vi "RT Main 9049.vi"() -> ()   [LabVIEW 2018]
doc: "This template is for the Queued Message Handler design pattern.\n\nThe Event Handling Loop generates messages based on user interface actions.\n\nThe Message Handling Loop processes messages generated by the Event Handling Loop, or by other messages. The messages are string values, so new messages can be added easily to the Message Cases case structure in the Message Handling Loop. Each message cluster can also provide an optional value for Message Data, which is a variant that can be converted to whatever message-specific data is required."
uses:
  support/Message Queue/Message Queue.lvlib
  Globals/Global - All RT Loop Stop.vi
  Globals/Global - Configuration Options.vi
  <vilib>/rvi/interface/nirviCloseFPGA/nirviCloseFPGA.xnode
  Globals/Global - RT Stream Connections.vi
  <vilib>/nisyscfg/nisyscfg.lvlib
  COMET  Extra Programs/Globals/Global - Monitoring Variables.vi
  controls/FPGA VI Reference 9049.ctl
  <vilib>/FPGAPlugInAG/Dynamic/niLvFpga_Close_Dynamic.vi
panel:
  out "error out":errorcluster
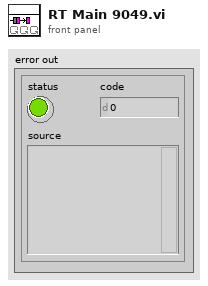
[diagram p1: front panel]
types:
  T1 = typedef "Acquisition and Logging Configuration.ctl" = cluster{"Samples per Read 9237":i32, "Number of Reads to Save":i32, "Data File Name 9222_9039_EXP":string, "TDMS Properties 9222":T2[], "Number of Channels 9237_9049_MAIN":i32, "Trigger - RMS Value":dbl, "Trigger - Channel":i32, "Trigger - Time (Minute)":i32, "Data Rate 9237":T3, "Number of Channels 9222_9039_EXP":i32, "Samples per Read 9222":i32, "Data Rate 9222":i32, "Channel Names 9222_9039_EXP":string[], "TDMS Properties 9237":T2[], "Data File Name 9237_9049":string, "Excitation Voltage":T4, "Data File Name 9222_9049_MAIN":string, "Number of Channels 9222_9049_MAIN":i32, "Channel Names 9222_9049_MAIN":string[], "Data File Name 9237_9039":string, "Channel Names 9237_9039_EXP":string[], "Channel Names 9237_9049_MAIN":string[], "Number of Channels 9237_9039_EXP":i32}
  T2 = typedef "TDMS Properties.ctl" = cluster{"Name":string, "Value":string}
  T3 = typedef "nicrio_cRIO-9237_DataRatesRing.ctl" = u8
  T4 = typedef "nicrio_cRIO-9237_ExcitationVoltageRing.ctl" = u8
  T5 = typedef "FPGA VI Reference 9049.ctl" = refnum<k20>
  T6 = typedef "Message Queue.lvlib/All Real-Time Message Queues Multi Queues.ctl" = cluster{"Message Handler":refnum<queue>, "Acquisition and Logging 9237":refnum<queue>, "Emergeny Stop for DCs":refnum<queue>, "LNG DC Commands":refnum<queue>, "LOX DC Commands":refnum<queue>, "NGV DC Commands":refnum<queue>, "Acquisition and Logging 9222":refnum<queue>, "Acquisition and Logging 9222_MAIN":refnum<queue>, "AUTO P&D":refnum<queue>, "Pressure Control":refnum<queue>}
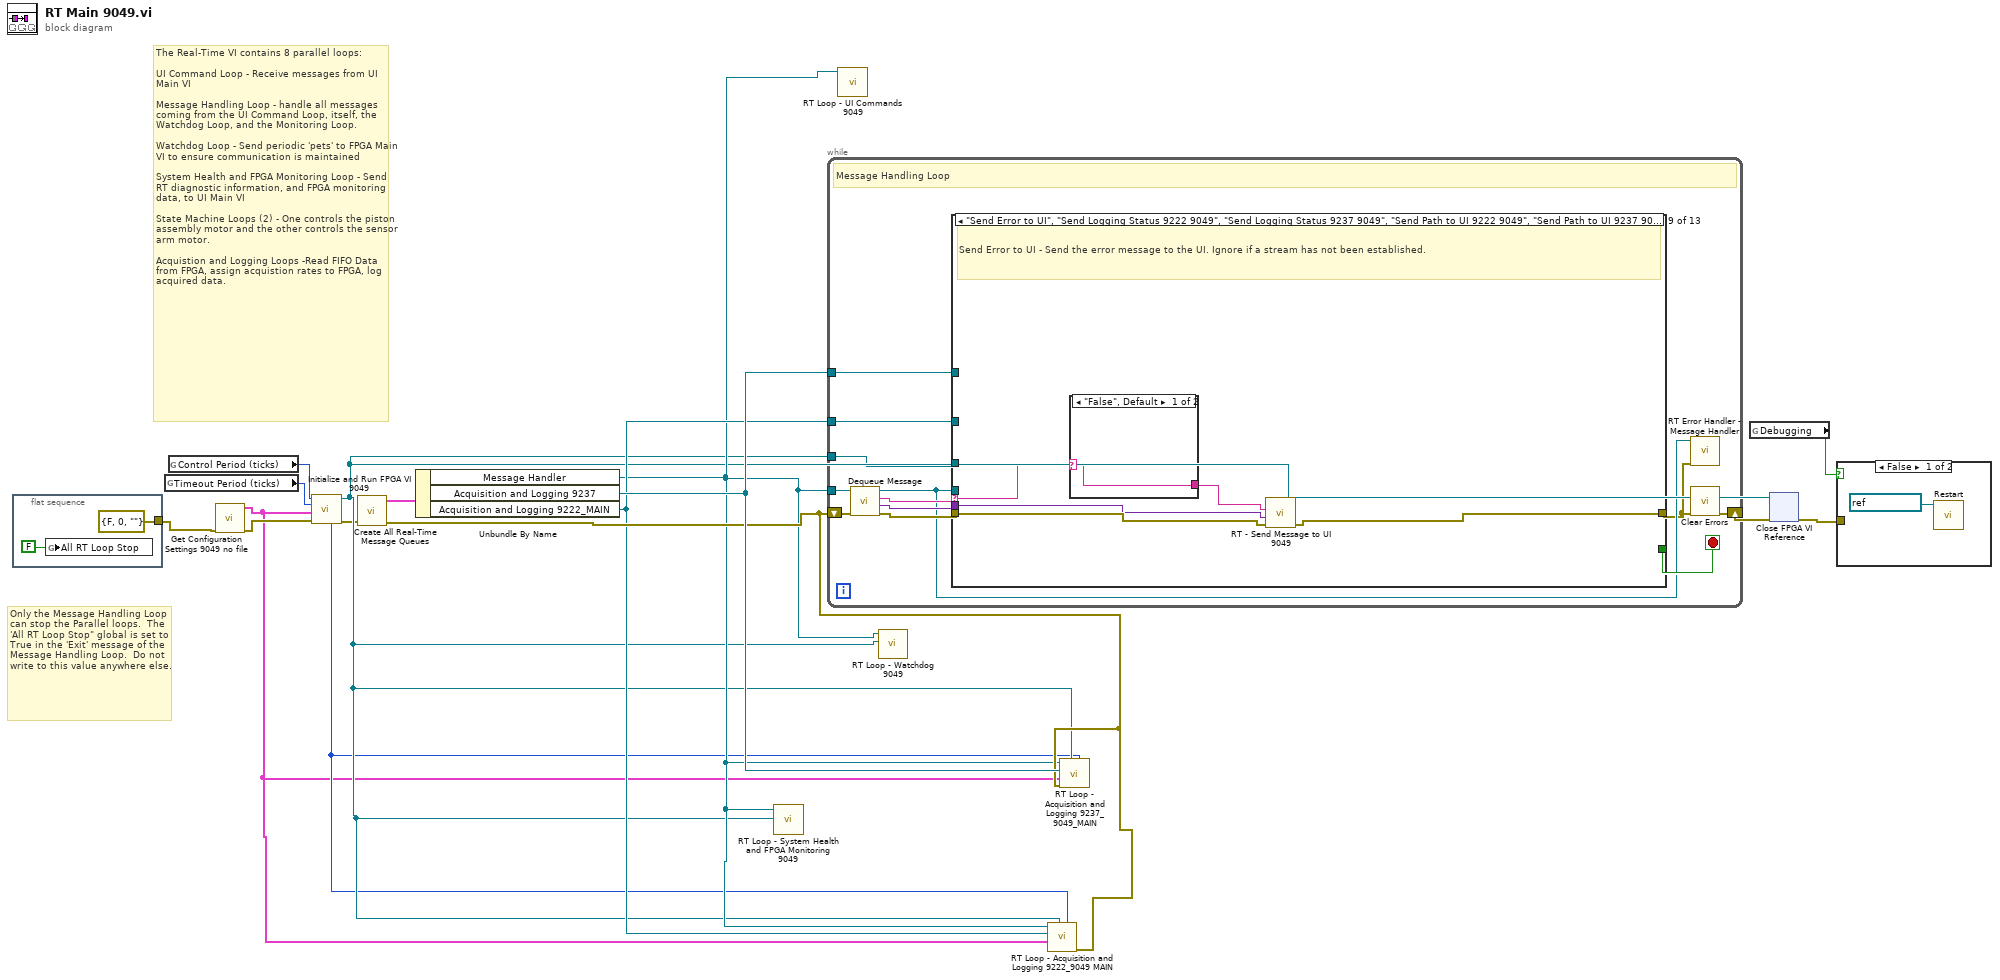
[diagram p0: block diagram]
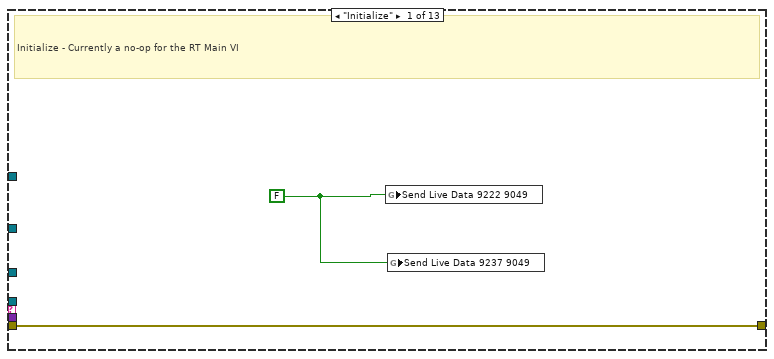
[diagram p3: hidden frame]
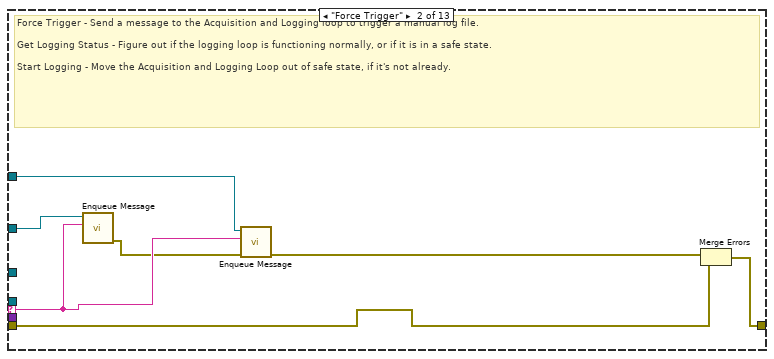
[diagram p4: hidden frame]
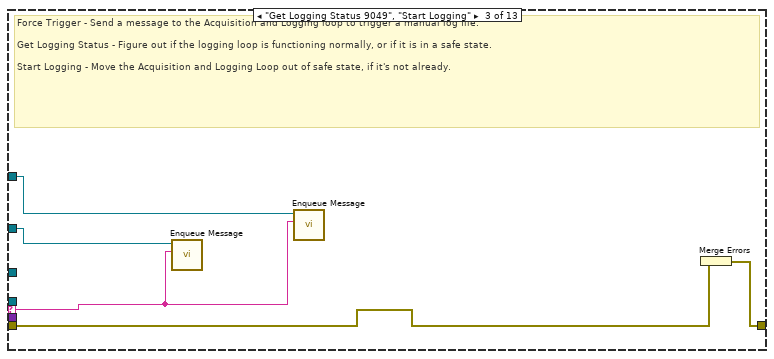
[diagram p5: hidden frame]
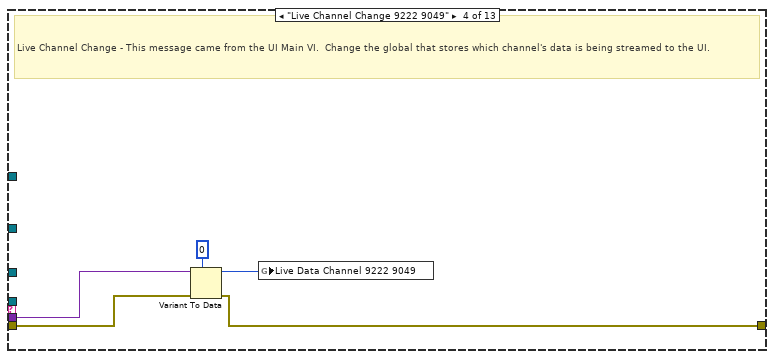
[diagram p6: hidden frame]
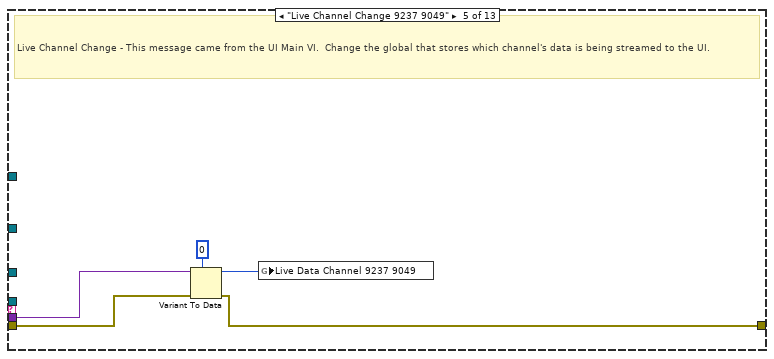
[diagram p7: hidden frame]
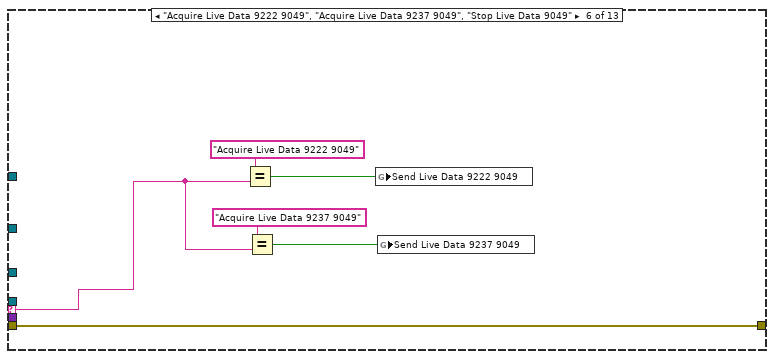
[diagram p8: hidden frame]
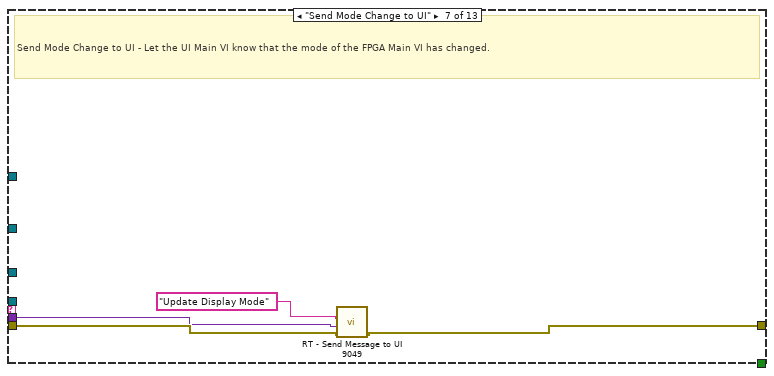
[diagram p9: hidden frame]
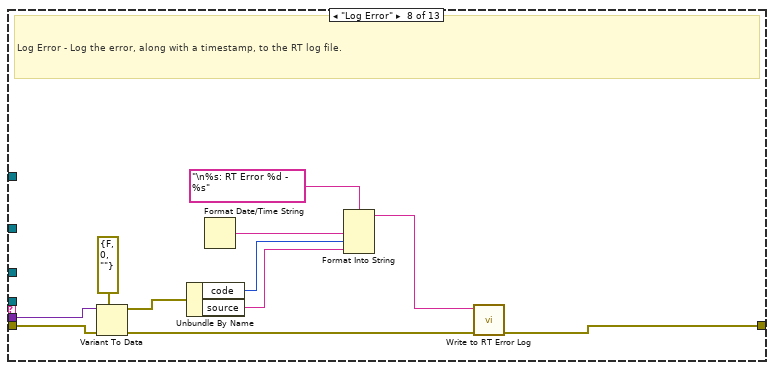
[diagram p10: hidden frame]
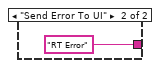
[diagram p11: hidden frame]
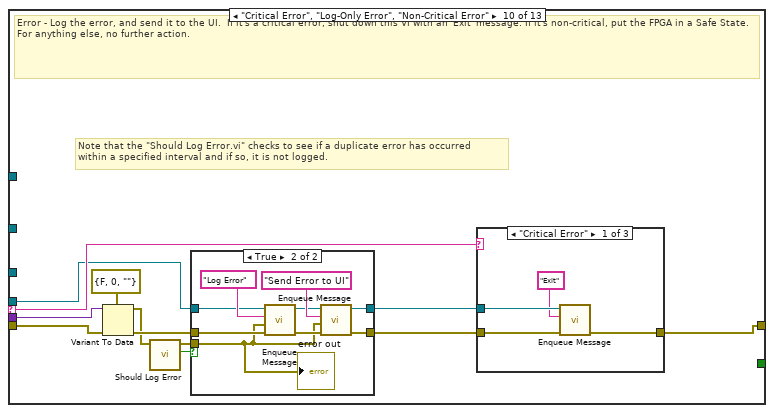
[diagram p12: hidden frame]
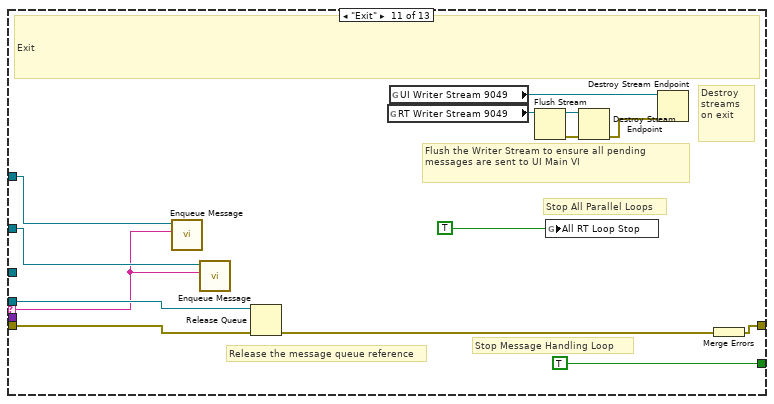
[diagram p16: hidden frame]
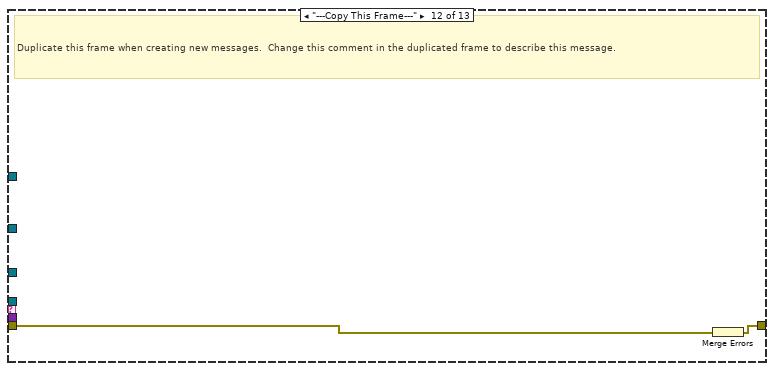
[diagram p17: hidden frame]
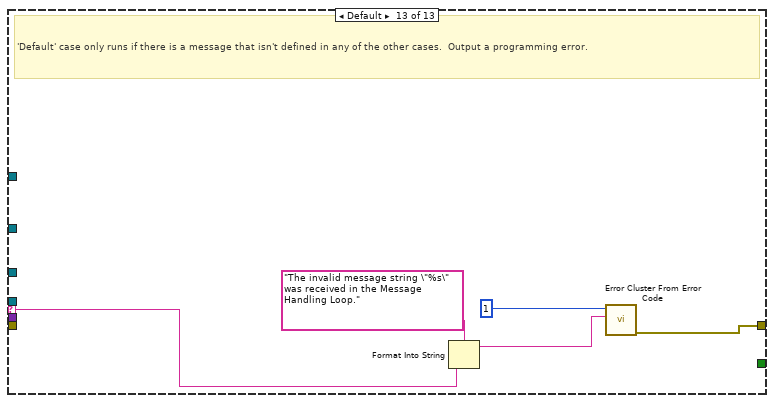
[diagram p18: hidden frame]
diagram:
  # "The Real-Time VI contains 8 parallel loops:\n\nUI Command Loop - Receive messages from UI Main VI\n\nMessage Handling Loop - handle all messages coming from the UI Command Loop, itself, the Watchdog Loop, and the Monitoring Loop.\n\nWatchdog Loop - Send periodic 'pets' to FPGA Main VI to ensure communication is maintained\n\nSystem Health and FPGA Monitoring Loop - Send RT diagnostic information, and FPGA monitoring data, to UI Main VI\n\nState Machine Loops (2) - One controls the piston assembly motor and the other controls the sensor arm motor.\n\nAcquistion and Logging Loops -Read FIFO Data from FPGA, assign acquistion rates to FPGA, log acquired data."
  # "Only the Message Handling Loop can stop the Parallel loops.  The 'All RT Loop Stop\" global is set to True in the 'Exit' message of the Message Handling Loop.  Do not write to this value anywhere else."
  n1 = flat-sequence {
    tunnel: [errorcluster {"status"=FALSE, "code"=0, "source"=""} ("error constant")] -> w12
    frame #0 {
      n2 = global write "Global - All RT Loop Stop.vi" "All RT Loop Stop"(FALSE) -> ()
    }
  }
  n3 = global read "Global - Configuration Options.vi" "Timeout Period (ticks)"() -> (w9:u64)
  n4 = global read "Global - Configuration Options.vi" "Control Period (ticks)"() -> (w8:u32)
  n5 = call "Get Configuration Settings 9049 no file.vi"("error in (no error)"=w12) -> ("error out"=w10:errorcluster, "Acquisition and Logging Configuration"=w2:T1)  [unwired: 9 in]
  n6 = call "Initialize and Run FPGA VI 9049.vi"("error in (no error)"=w10, "Acquisition and Logging Configuration"=w2, "Timeout Period (ticks)"=w9, "Control Period (ticks)"=w8) -> ("error out"=w1:errorcluster, "FPGA VI Reference 9049"=w4:T5, "Total Buffer Size 9222"=w3:i32)  [unwired: 5 in]
  n7 = call "Create All Real-Time Message Queues.vi"("error in (no error)"=w1) -> ("error out"=w7:errorcluster, "Message Queues out"=w13:T6)  [unwired: 9 in]
  n8 = Unbundle By Name(w13) -> ("Message Handler"=w5:refnum<queue>, "Acquisition and Logging 9237"=w11:refnum<queue>, "Acquisition and Logging 9222_MAIN"=w6:refnum<queue>)
  n9 = call "RT Loop - System Health and FPGA Monitoring 9049.vi"("FPGA VI Reference 9049"=w4, "Message Queue"=w5) -> ()  [unwired: 10 in]
  n10 = while {
    tunnel: w5 -> [w25]
    shift-right: [w22] -> w16
    shift-left: w7 -> [w29]
    tunnel: w4 -> [w24]
    tunnel: w11 -> [w20]
    tunnel: w6 -> [w19]
    stop <- w30 stop-if-true
    # "Message Handling Loop"
    n11 = call "Dequeue Message.vi"("error in (no error)"=w29, "Message Queue"=w25) -> ("error out"=w28:errorcluster, "Message Data"=w26:variant, "Message"=w27:string, "dup Message Queue"=w23:refnum<queue>)  [unwired: 6 in]
    n12 = case "Message Cases" shown="\"Send Error to UI\", \"Send Logging Status 9222 9049\", \"Send Logging Status 9237 9049\", \"Send Path to UI 9222 9049\", \"Send Path to UI 9237 9049\"" w27 {
      selector: w27 -> [_ w35 w41 _ _ w55 _ _ w80 w92 w112 _ w131]
      tunnel: w23 -> [_ _ _ _ _ _ _ _ _ w86 w125 _ _]
      tunnel: w28 -> [w32 w37 w43 w47 w52 w60 w63 w75 w78 w90 w121 w127 _]
      tunnel: [w32 w39 w44 w46 w51 w60 w64 w66 w79 w91 w122 w126 w129] -> w21
      tunnel: [_ _ _ _ _ _ _ _ _ _ TRUE _ _] -> w30
      tunnel: w26 -> [_ _ _ w45 w50 _ w62 w74 w77 w89 _ _ _]
      tunnel: w24 -> [_ _ _ _ _ _ _ _ _ _ _ _ _]
      tunnel: w20 -> [_ w38 w42 _ _ _ _ _ _ _ w114 _ _]
      tunnel: w19 -> [_ w36 w40 _ _ _ _ _ _ _ w113 _ _]
      frame "Initialize" {
        w31 = FALSE ("Send Live Data 9222 9049")
        # "Initialize - Currently a no-op for the RT Main VI"
        n13 = global write "Global - Monitoring Variables.vi" "Send Live Data 9222 9049"(w31) -> ()
        n14 = global write "Global - Monitoring Variables.vi" "Send Live Data 9237 9049"(w31) -> ()
      }
      frame "Force Trigger" {
        # "Force Trigger - Send a message to the Acquisition and Logging loop to trigger a manual log file.\n\nGet Logging Status - Figure out if the logging loop is functioning normally, or if it is in a safe state.\n\nStart Logging - Move the Acquisition and Logging Loop out of safe state, if it's not already."
        n15 = call "Enqueue Message.vi"("Message"=w35, "Message Queue"=w36) -> ("error out"=w34:errorcluster)  [unwired: 8 in, 1 out]
        n16 = call "Enqueue Message.vi"("error in (no error)"=w34, "Message"=w35, "Message Queue"=w38) -> ("error out"=w33:errorcluster)  [unwired: 7 in, 1 out]
        n17 = Merge Errors(w33, w37) -> (w39:errorcluster)
      }
      frame "Get Logging Status 9049", "Start Logging" {
        # "Force Trigger - Send a message to the Acquisition and Logging loop to trigger a manual log file.\n\nGet Logging Status - Figure out if the logging loop is functioning normally, or if it is in a safe state.\n\nStart Logging - Move the Acquisition and Logging Loop out of safe state, if it's not already."
        n18 = call "Enqueue Message.vi"("Message"=w41, "Message Queue"=w40) -> ()  [unwired: 8 in, 2 out]
        n19 = call "Enqueue Message.vi"("Message"=w41, "Message Queue"=w42) -> ()  [unwired: 8 in, 2 out]
        n20 = Merge Errors(w43) -> (w44:errorcluster)
      }
      frame "Live Channel Change 9222 9049" {
        # "Live Channel Change - This message came from the UI Main VI.  Change the global that stores which channel's data is being streamed to the UI."
        n21 = Variant To Data(error in=w47, type=u32 0, Variant=w45) -> (data=w49:u32, error out=w46:errorcluster)
        n22 = global write "Global - Monitoring Variables.vi" "Live Data Channel 9222 9049"(w49) -> ()
      }
      frame "Live Channel Change 9237 9049" {
        # "Live Channel Change - This message came from the UI Main VI.  Change the global that stores which channel's data is being streamed to the UI."
        n23 = Variant To Data(error in=w52, type=u32 0, Variant=w50) -> (data=w54:u32, error out=w51:errorcluster)
        n24 = global write "Global - Monitoring Variables.vi" "Live Data Channel 9237 9049"(w54) -> ()
      }
      frame "Acquire Live Data 9222 9049", "Acquire Live Data 9237 9049", "Stop Live Data 9049" {
        n25 = Equal?(x="Acquire Live Data 9222 9049", y=w55) -> (x = y?=w58:bool)
        n26 = Equal?(x="Acquire Live Data 9237 9049", y=w55) -> (x = y?=w57:bool)
        n27 = global write "Global - Monitoring Variables.vi" "Send Live Data 9222 9049"(w58) -> ()
        n28 = global write "Global - Monitoring Variables.vi" "Send Live Data 9237 9049"(w57) -> ()
      }
      frame "Send Mode Change to UI" {
        # "Send Mode Change to UI - Let the UI Main VI know that the mode of the FPGA Main VI has changed."
        n29 = call "RT - Send Message to UI 9049.vi"("error in (no error)"=w63, "Message Data"=w62, "Message"="Update Display Mode") -> ("error out"=w64:errorcluster)  [unwired: 8 in]
      }
      frame "Log Error" {
        # "Log Error - Log the error, along with a timestamp, to the RT log file."
        n30 = Variant To Data(error in=w75, type=errorcluster {"status"=FALSE, "code"=0, "source"=""} ("error constant"), Variant=w74) -> (data=w69:errorcluster, error out=w72:errorcluster)
        n31 = Unbundle By Name(w69) -> ("code"=w68:i32, "source"=w67:string)
        n32 = Format Date/Time String() -> (date/time string=w70:string)  [unwired: 3 in]
        n33 = Format Into String(format string="\n%s: RT Error %d - %s", w70, w68, w67) -> (resulting string=w65:string)  [unwired: 2 in, 1 out]
        n34 = call "Write to RT Error Log.vi"("error in (no error)"=w72, "Log Entry"=w65) -> ("error out"=w66:errorcluster)  [unwired: 9 in]
      }
      frame "Send Error to UI", "Send Logging Status 9222 9049", "Send Logging Status 9237 9049", "Send Path to UI 9222 9049", "Send Path to UI 9237 9049" {
        # "Send Error to UI - Send the error message to the UI. Ignore if a stream has not been established."
        n35 = case shown="\"False\", Default" w80 {
          selector: w80 -> [w81 _]
          tunnel: [w81 "RT Error" ("Message")] -> w76
          frame "False", Default {
          }
          frame "Send Error To UI" {
          }
        }
        n36 = call "RT - Send Message to UI 9049.vi"("error in (no error)"=w78, "Message Data"=w77, "Message"=w76) -> ("error out"=w79:errorcluster)  [unwired: 8 in]
      }
      frame "Critical Error", "Log-Only Error", "Non-Critical Error" {
        # "Note that the \"Should Log Error.vi\" checks to see if a duplicate error has occurred \nwithin a specified interval and if so, it is not logged."
        # "Error - Log the error, and send it to the UI.  If it's a critical error, shut down this VI with an 'Exit' message. If it's non-critical, put the FPGA in a Safe State. For anything else, no further action."
        n37 = Variant To Data(error in=w90, type=errorcluster {"status"=FALSE, "code"=0, "source"=""} ("error out"), Variant=w89) -> (data=w83:errorcluster, error out=w87:errorcluster)
        n38 = call "Should Log Error.vi"("error to report"=w83) -> ("Should Log Error?"=w85:bool, "dup error to report"=w84:errorcluster)  [unwired: 9 in]
        n39 = case shown="True" w85 {
          tunnel: [w96 w103] -> w94
          tunnel: [w95 w102] -> w93
          tunnel: w86 -> [w95 w101]
          tunnel: w87 -> [w96 w98]
          tunnel: w84 -> [_ w97]
          frame False {
          }
          frame True {
            n40 = call "Enqueue Message.vi"("error in (no error)"=w98, "Message Data"=w97, "Message"="Log Error", "Message Queue"=w101) -> ("error out"=w99:errorcluster, "dup Message Queue"=w100:refnum<queue>)  [unwired: 6 in]
            n41 = call "Enqueue Message.vi"("error in (no error)"=w99, "Message Data"=w97, "Message"="Send Error to UI", "Message Queue"=w100) -> ("error out"=w103:errorcluster, "dup Message Queue"=w102:refnum<queue>)  [unwired: 6 in]
            "error out" <- w97
          }
        }
        n42 = case shown="\"Critical Error\"" w92 {
          tunnel: w94 -> [w109 w110 w111]
          tunnel: w93 -> [w107 _ _]
          tunnel: [w108 w110 w111] -> w91
          frame "Critical Error" {
            n43 = call "Enqueue Message.vi"("error in (no error)"=w109, "Message"="Exit", "Message Queue"=w107) -> ("error out"=w108:errorcluster)  [unwired: 7 in, 1 out]
          }
          frame "Non-Critical Error" {
          }
          frame Default {
          }
        }
      }
      frame "Exit" {
        # "Flush the Writer Stream to ensure all pending messages are sent to UI Main VI"
        # "Destroy streams on exit"
        # "Stop Message Handling Loop"
        # "Stop All Parallel Loops"
        # "Release the message queue reference"
        # "Exit"
        n44 = call "Enqueue Message.vi"("Message"=w112, "Message Queue"=w114) -> ()  [unwired: 8 in, 2 out]
        n45 = call "Enqueue Message.vi"("Message"=w112, "Message Queue"=w113) -> ()  [unwired: 8 in, 2 out]
        n46 = Release Queue(queue=w125, error in (no error)=w121) -> (error out=w123:errorcluster)  [unwired: 1 in, 2 out]
        n47 = global read "Global - RT Stream Connections.vi" "RT Writer Stream 9049"() -> (w117:refnum<k21>)
        n48 = global read "Global - RT Stream Connections.vi" "UI Writer Stream 9049"() -> (w119:refnum<k21>)
        n49 = Flush Stream(11:w117) -> (0:w115:errorcluster, 3:w116:refnum<k21>)  [unwired: 3 in, 1 out]
        n50 = global write "Global - All RT Loop Stop.vi" "All RT Loop Stop"(TRUE ("Stop Monitoring Loops")) -> ()
        n51 = Destroy Stream Endpoint(8:w115, 11:w116) -> (0:w118:errorcluster)
        n52 = Destroy Stream Endpoint(8:w118, 11:w119) -> ()  [unwired: 1 out]
        n53 = Merge Errors(w123) -> (w122:errorcluster)
      }
      frame "---Copy This Frame---" {
        # "Duplicate this frame when creating new messages.  Change this comment in the duplicated frame to describe this message."
        n54 = Merge Errors(w127) -> (w126:errorcluster)
      }
      frame Default {
        # "'Default' case only runs if there is a message that isn't defined in any of the other cases.  Output a programming error."
        n55 = Format Into String(format string="The invalid message string \"%s\" was received in the Message Handling Loop." ("Unknown Message Error Text"), w131) -> (resulting string=w128:string)  [unwired: 2 in, 1 out]
        n56 = call <vilib>:"Error Cluster From Error Code.vi"("error message (\"\")"=w128, "error code (0)"=1) -> ("error out"=w129:errorcluster)  [unwired: 7 in]
      }
    }
    n57 = call "RT Error Handler - Message Handler.vi"("error in (no error)"=w21, "Message Queue"=w23) -> ()  [unwired: 9 in, 1 out]
    n58 = call <vilib>:"Clear Errors.vi"("error in (no error)"=w21) -> ("error out"=w22:errorcluster)  [unwired: 5 in, 1 out]
  }
  n59 = call "RT Loop - UI Commands 9049.vi"("Message Queue"=w5) -> ()  [unwired: 11 in]
  n60 = call "RT Loop - Watchdog 9049.vi"("FPGA VI Reference 2"=w4, "Message Queue"=w5) -> ()  [unwired: 10 in]
  n61 = call "RT Loop - Acquisition and Logging 9222_9049 MAIN.vi"("Total Buffer Size"=w3, "FPGA VI Reference 9049"=w4, "error in (no error)"=w7, "Acquisition and Logging Configuration"=w2, "Acquisition and Logging Queue"=w6, "Message Queue"=w5) -> ()  [unwired: 6 in]
  n62 = call "RT Loop - Acquisition and Logging 9237_9049_MAIN.vi"("Total Buffer Size"=w3, "FPGA VI Reference 9049"=w4, "error in (no error)"=w7, "Acquisition and Logging Configuration"=w2, "Acquisition and Logging Queue"=w11, "Message Queue"=w5) -> ()  [unwired: 6 in]
  n63 = global read "Global - Configuration Options.vi" "Debugging"() -> (w14:bool)
  n64 = xnode "Close FPGA VI Reference"("FPGA VI Reference In"=w4, "error in"=w16) -> ("error out"=w15:errorcluster)
  n65 = case shown="False" w14 {
    tunnel: w15 -> [_ _]
    frame False {
      n66 = call <vilib>:"Restart.vi"("Session in"=refnum<k21> "localhost" ("session in")) -> ()  [unwired: 8 in, 3 out]
    }
    frame True {
    }
  }
